vi "Game ID FG.vi"() -> (3 "Game ID":u16)   [LabVIEW 2020, in "SquareBattle.lvlib" / "Game.lvclass"]
uses:
  Game.lvclass
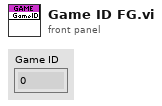
[diagram p1: front panel]
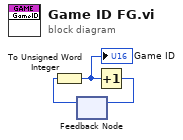
[diagram p0: block diagram]
diagram:
  n1 = feedback #1() -> (w1:u16)  [unwired: 1 in]
  n2 = To Unsigned Word Integer(number=w1) -> (unsigned 16bit integer=w3:u16)
  "Game ID" <- w3
  n3 = Increment(x=w3) -> (x+1=w2:u16)
  n4 = feedback-in #1(w2) -> ()
